vi "Sr530 Read Param.vi"(0 "Ressource VISA":refnum<visa-resource-name>="GPIB0::8::INSTR", 5 "error in (no error)":errorcluster) -> (14 "Ressource VISA Out":refnum<visa-resource-name>="GPIB0::8::INSTR", 15 "LockInPar":T1={"BandFilter"=FALSE, "LineFilter1x"=FALSE, "LineFilter2x"=FALSE, "Expand Ch1"=FALSE, "Expand Ch2"=FALSE, "Sensitivity"=1, "Pre Time"=1, "Post Time"=0, "Dynamic Res."=0, "Reference Trigger"=0, "Channels Settings"=0, "Frequency"=0.0} caption="Lock-In Parameters" {"Channels Settings" items=["X, Y", "X Offset, Y Offset", "R, Teta", "R Offset, Teta", "X Noise, Y Noise", "X5 (D/A), X6 (D/A)"]; "Reference Trigger" items=["Positive", "Symmetric", "Negative"]; "Post Time" items=["None", "0.1 s", "1 s"]; "Pre Time" items=["1 ms"=1, "3 ms"=2, "10 ms"=3, "30 ms"=4, "100 ms"=5, "300 ms"=6, "1 s"=7, "3 s"=8, "10 s"=9, "30 s"=10, "100 s"=11]; "Sensitivity" items=["10 nV"=1, "20 nV"=2, "50 nV"=3, "100 nV"=4, "200 nV"=5, "500 nV"=6, "1 µV"=7, "2 µV"=8, "5 µV"=9, "10 µV"=10, "20 µV"=11, "50 µV"=12, "100µV"=13, "200 µV"=14, "500µV"=15, "1 mV"=16, "2 mV"=17, "5 mV"=18, "10 mV"=19, "20 mV"=20, "50 mV"=21, "100 mV"=22]; "Dynamic Res." items=["Low", "Normal", "High"]}, 16 "Params":string, 19 "error out":errorcluster)   [LabVIEW 2019]
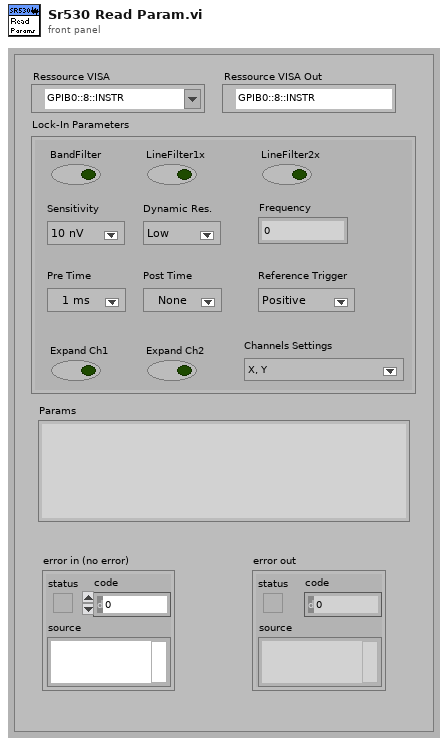
[diagram p1: front panel]
types:
  T1 = cluster{"BandFilter":bool, "LineFilter1x":bool, "LineFilter2x":bool, "Expand Ch1":bool, "Expand Ch2":bool, "Sensitivity":u16, "Pre Time":u16, "Post Time":u16, "Dynamic Res.":u16, "Reference Trigger":u16, "Channels Settings":u16, "Frequency":dbl}
  T2 = enum16{"BandPass Filter", "Dynamic Reserve", "Expand", "Frequency", "Ref Trig", "Ch Settings", "Gain", "Notch Filter", "Time Constant", "End"}
  T3 = cluster{"BandFilter":bool, "LineFilter1x":bool, "LineFilter2x":bool, "Expand Ch1":bool, "Expand Ch2":bool, "Sensitivity":u16, "Dynamic Reserve":u16, "Pre Time":u16, "Post Time":u16, "Reference Trigger":u16, "Channels Settings":u16, "Frequency":dbl}
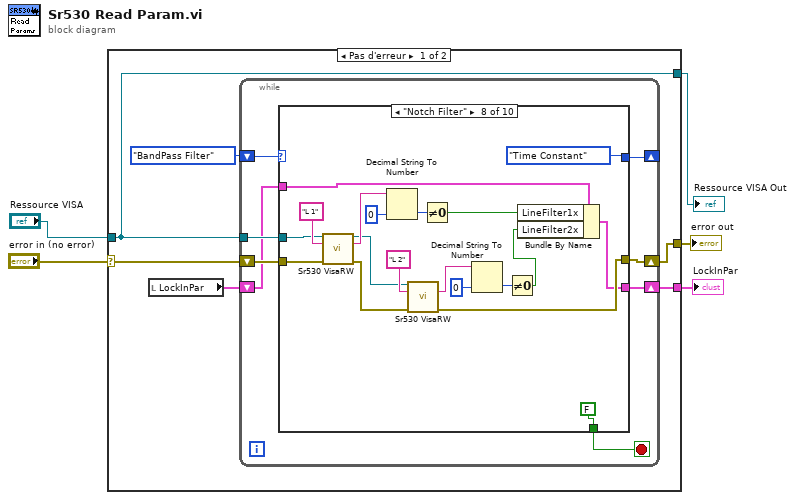
[diagram p0: block diagram]
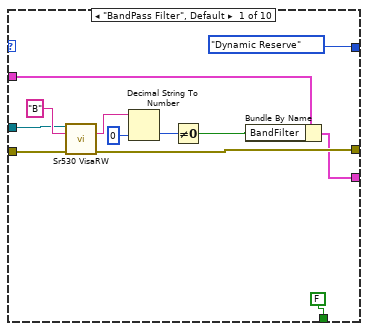
[diagram p2: hidden frame]
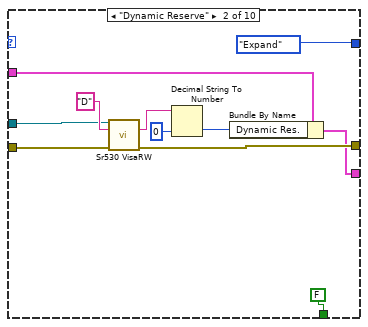
[diagram p3: hidden frame]
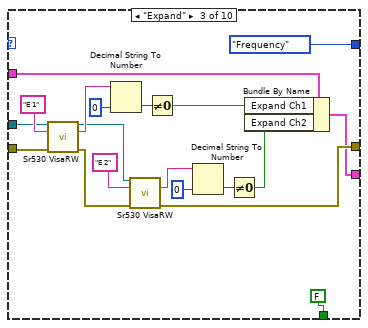
[diagram p4: hidden frame]
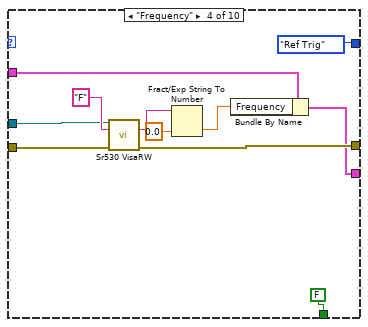
[diagram p5: hidden frame]
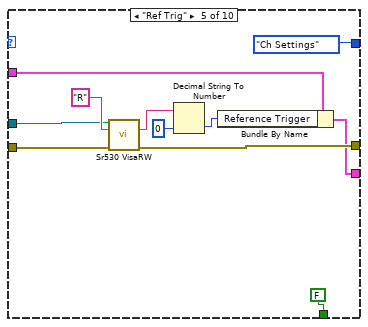
[diagram p6: hidden frame]
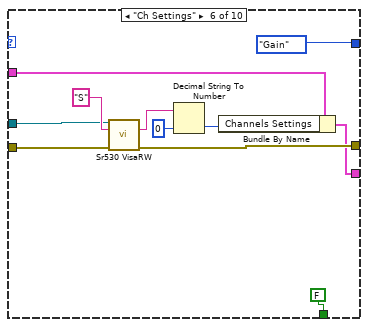
[diagram p7: hidden frame]
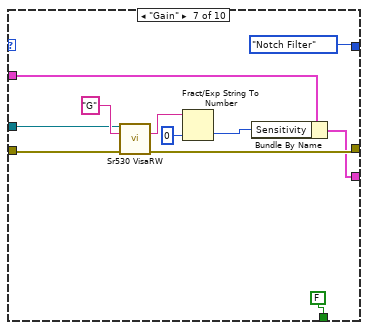
[diagram p8: hidden frame]
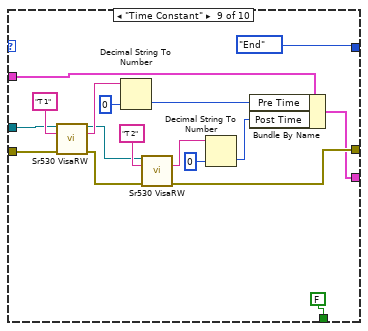
[diagram p9: hidden frame]
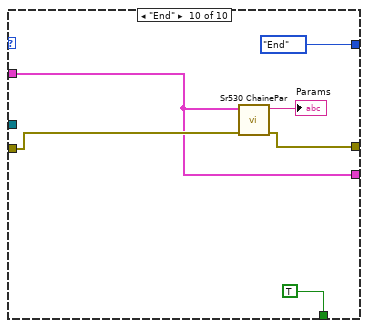
[diagram p10: hidden frame]
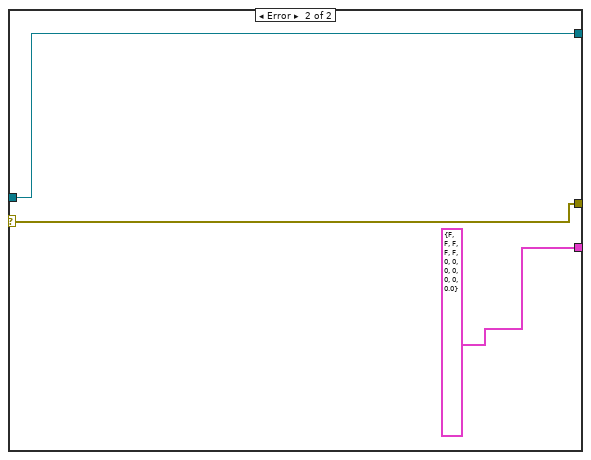
[diagram p11: hidden frame]
diagram:
  n1 = case shown="Pas d'erreur" "error in (no error)" {
    selector: "error in (no error)" -> [w10 w150]
    tunnel: [w11 w150] -> w4
    tunnel: [w8 w149] -> w3
    tunnel: "Ressource VISA" -> [w8 w149]
    tunnel: [w7 T3 {"BandFilter"=FALSE, "LineFilter1x"=FALSE, "LineFilter2x"=FALSE, "Expand Ch1"=FALSE, "Expand Ch2"=FALSE, "Sensitivity"=0, "Dynamic Reserve"=0, "Pre Time"=0, "Post Time"=0, "Reference Trigger"=0, "Channels Settings"=0, "Frequency"=0.0} ("LockInPar")] -> w1
    frame No Error {
      n2 = local read "LockInPar"() -> (w6:T1)
      n3 = while {
        shift-right: [w15] -> _
        shift-left: T2."BandPass Filter" -> [w19]
        shift-right: [w17] -> w11
        shift-left: w10 -> [w18]
        tunnel: w8 -> [w16]
        shift-right: [w13] -> w7
        shift-left: w6 -> [w12]
        stop <- w14 stop-if-true
        n4 = case shown="\"Notch Filter\"" w19 {
          tunnel: w18 -> [w30 w41 w57 w71 w82 w93 w102 w123 w132 w145]
          tunnel: [w29 w40 w49 w70 w81 w92 w100 w112 w133 w143] -> w17
          tunnel: w16 -> [w28 w39 w58 w69 w80 w91 w101 w122 w131 _]
          tunnel: [T2."Dynamic Reserve" T2."Expand" T2."Frequency" T2."Ref Trig" T2."Ch Settings" T2."Gain" T2."Notch Filter" T2."Time Constant" T2."End" T2."End"] -> w15
          tunnel: [FALSE FALSE FALSE FALSE FALSE FALSE FALSE FALSE FALSE TRUE] -> w14
          tunnel: w12 -> [w22 w33 w43 w64 w74 w84 w95 w107 w127 w144]
          tunnel: [w20 w34 w44 w63 w73 w85 w96 w106 w125 w144] -> w13
          frame "BandPass Filter", Default {
            n5 = call <userlib>:"Sr530 VisaRW.vi"("VISA Rsrc"=w28, "ChaineCom"="B", "error in (no error)"=w30) -> ("ChaineRep"=w27:string, "error out"=w29:errorcluster)  [unwired: 7 in, 4 out]
            n6 = Decimal String To Number(string=w27, default (0L)=u8 0 ("valeur par défaut (0 I32)")) -> (number=w25:u8)  [unwired: 1 in, 1 out]
            n7 = Not Equal To 0?(x=w25) -> (x != 0?=w21:bool)
            n8 = Bundle By Name(cluster=w22, "BandFilter"=w21) -> (w20:T1)
          }
          frame "Dynamic Reserve" {
            n9 = call <userlib>:"Sr530 VisaRW.vi"("VISA Rsrc"=w39, "ChaineCom"="D", "error in (no error)"=w41) -> ("ChaineRep"=w38:string, "error out"=w40:errorcluster)  [unwired: 7 in, 4 out]
            n10 = Decimal String To Number(string=w38, default (0L)=u16 0 ("valeur par défaut (0 I32)")) -> (number=w32:u16)  [unwired: 1 in, 1 out]
            n11 = Bundle By Name(cluster=w33, "Dynamic Res."=w32) -> (w34:T1)
          }
          frame "Expand" {
            n12 = call <userlib>:"Sr530 VisaRW.vi"("VISA Rsrc"=w58, "ChaineCom"="E 1", "error in (no error)"=w57) -> ("VISA Rsrc Out"=w50:refnum<visa-resource-name>, "ChaineRep"=w60:string, "error out"=w51:errorcluster)  [unwired: 7 in, 3 out]
            n13 = Decimal String To Number(string=w60, default (0L)=u16 0 ("valeur par défaut (0 I32)")) -> (number=w56:u16)  [unwired: 1 in, 1 out]
            n14 = call <userlib>:"Sr530 VisaRW.vi"("VISA Rsrc"=w50, "ChaineCom"="E 2", "error in (no error)"=w51) -> ("ChaineRep"=w53:string, "error out"=w49:errorcluster)  [unwired: 7 in, 4 out]
            n15 = Not Equal To 0?(x=w56) -> (x != 0?=w45:bool)
            n16 = Decimal String To Number(string=w53, default (0L)=u16 0 ("valeur par défaut (0 I32)")) -> (number=w55:u16)  [unwired: 1 in, 1 out]
            n17 = Not Equal To 0?(x=w55) -> (x != 0?=w46:bool)
            n18 = Bundle By Name(cluster=w43, "Expand Ch1"=w45, "Expand Ch2"=w46) -> (w44:T1)
          }
          frame "Frequency" {
            n19 = call <userlib>:"Sr530 VisaRW.vi"("VISA Rsrc"=w69, "ChaineCom"="F", "error in (no error)"=w71) -> ("ChaineRep"=w68:string, "error out"=w70:errorcluster)  [unwired: 7 in, 4 out]
            n20 = Fract/Exp String To Number(string=w68, default (0 dbl)=0.0 ("valeur par défaut (0 I32)")) -> (number=w62:dbl)  [unwired: 2 in, 1 out]
            n21 = Bundle By Name(cluster=w64, "Frequency"=w62) -> (w63:T1)
          }
          frame "Ref Trig" {
            n22 = call <userlib>:"Sr530 VisaRW.vi"("VISA Rsrc"=w80, "ChaineCom"="R", "error in (no error)"=w82) -> ("ChaineRep"=w76:string, "error out"=w81:errorcluster)  [unwired: 7 in, 4 out]
            n23 = Decimal String To Number(string=w76, default (0L)=u16 0 ("valeur par défaut (0 I32)")) -> (number=w75:u16)  [unwired: 1 in, 1 out]
            n24 = Bundle By Name(cluster=w74, "Reference Trigger"=w75) -> (w73:T1)
          }
          frame "Ch Settings" {
            n25 = call <userlib>:"Sr530 VisaRW.vi"("VISA Rsrc"=w91, "ChaineCom"="S", "error in (no error)"=w93) -> ("ChaineRep"=w87:string, "error out"=w92:errorcluster)  [unwired: 7 in, 4 out]
            n26 = Decimal String To Number(string=w87, default (0L)=u16 0 ("valeur par défaut (0 I32)")) -> (number=w86:u16)  [unwired: 1 in, 1 out]
            n27 = Bundle By Name(cluster=w84, "Channels Settings"=w86) -> (w85:T1)
          }
          frame "Gain" {
            n28 = call <userlib>:"Sr530 VisaRW.vi"("VISA Rsrc"=w101, "ChaineCom"="G", "error in (no error)"=w102) -> ("ChaineRep"=w104:string, "error out"=w100:errorcluster)  [unwired: 7 in, 4 out]
            n29 = Fract/Exp String To Number(string=w104, default (0 dbl)=u16 0 ("valeur par défaut (0 I32)")) -> (number=w97:u16)  [unwired: 2 in, 1 out]
            n30 = Bundle By Name(cluster=w95, "Sensitivity"=w97) -> (w96:T1)
          }
          frame "Notch Filter" {
            n31 = call <userlib>:"Sr530 VisaRW.vi"("VISA Rsrc"=w122, "ChaineCom"="L 1", "error in (no error)"=w123) -> ("VISA Rsrc Out"=w114:refnum<visa-resource-name>, "ChaineRep"=w121:string, "error out"=w113:errorcluster)  [unwired: 7 in, 3 out]
            n32 = Decimal String To Number(string=w121, default (0L)=u8 0 ("valeur par défaut (0 I32)")) -> (number=w120:u8)  [unwired: 1 in, 1 out]
            n33 = call <userlib>:"Sr530 VisaRW.vi"("VISA Rsrc"=w114, "ChaineCom"="L 2", "error in (no error)"=w113) -> ("ChaineRep"=w116:string, "error out"=w112:errorcluster)  [unwired: 7 in, 4 out]
            n34 = Not Equal To 0?(x=w120) -> (x != 0?=w108:bool)
            n35 = Decimal String To Number(string=w116, default (0L)=u8 0 ("valeur par défaut (0 I32)")) -> (number=w117:u8)  [unwired: 1 in, 1 out]
            n36 = Not Equal To 0?(x=w117) -> (x != 0?=w109:bool)
            n37 = Bundle By Name(cluster=w107, "LineFilter1x"=w108, "LineFilter2x"=w109) -> (w106:T1)
          }
          frame "Time Constant" {
            n38 = call <userlib>:"Sr530 VisaRW.vi"("VISA Rsrc"=w131, "ChaineCom"="T 1", "error in (no error)"=w132) -> ("VISA Rsrc Out"=w135:refnum<visa-resource-name>, "ChaineRep"=w140:string, "error out"=w134:errorcluster)  [unwired: 7 in, 3 out]
            n39 = Decimal String To Number(string=w140, default (0L)=u16 0 ("valeur par défaut (0 I32)")) -> (number=w128:u16)  [unwired: 1 in, 1 out]
            n40 = call <userlib>:"Sr530 VisaRW.vi"("VISA Rsrc"=w135, "ChaineCom"="T 2", "error in (no error)"=w134) -> ("ChaineRep"=w137:string, "error out"=w133:errorcluster)  [unwired: 7 in, 4 out]
            n41 = Decimal String To Number(string=w137, default (0L)=u16 0 ("valeur par défaut (0 I32)")) -> (number=w126:u16)  [unwired: 1 in, 1 out]
            n42 = Bundle By Name(cluster=w127, "Pre Time"=w128, "Post Time"=w126) -> (w125:T1)
          }
          frame "End" {
            n43 = call "Sr530 ChaînePar.vi"("entrée d'erreur (pas d'erreur)"=w145, "LockInPar"=w144) -> ("sortie d'erreur"=w143:errorcluster, "Chaîne"=→"Params":string)  [unwired: 8 in]
          }
        }
      }
    }
    frame Error {
    }
  }
  "error out" <- w4
  "Ressource VISA Out" <- w3
  "LockInPar" <- w1
